vi "String Builder.vi"(9 "Omega":dbl, 10 "damping":dbl, 11 "A":dbl) -> (1 "a(t) string":string, 2 "v(t) string":string, 3 "x(t) string":string)   [LabVIEW 2019]
panel:
  out "Omega String":string
  out "damping string":string
  out "A string":string
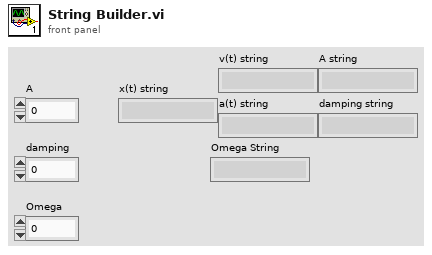
[diagram p1: front panel]
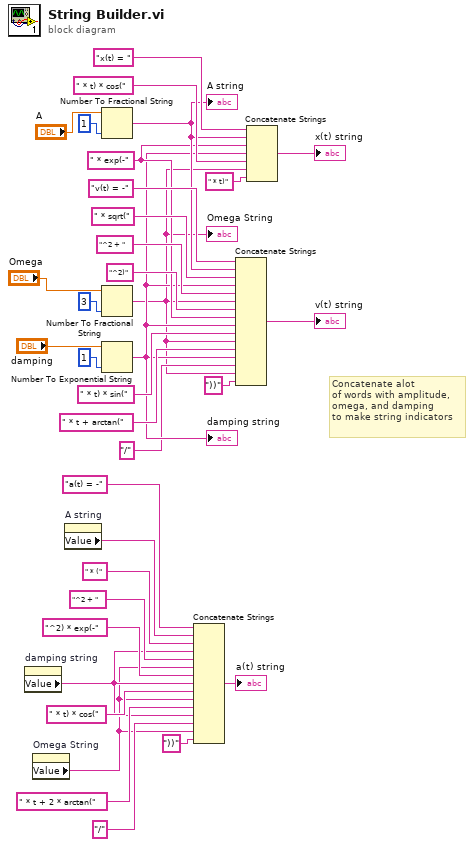
[diagram p0: block diagram]
diagram:
  w20 = " * exp(-"
  # "Concatenate alot\nof words with amplitude,\nomega, and damping\nto make string indicators"
  n1 = property on="damping string" class="Str"() -> ("Value"=w5:string)  [unwired: 2 in, 2 out]
  n2 = property on="Omega String" class="Str"() -> ("Value"=w3:string)  [unwired: 2 in, 2 out]
  n3 = property on="A string" class="Str"() -> ("Value"=w11:string)  [unwired: 2 in, 2 out]
  n4 = Number To Fractional String(number="A", precision (6)=i16 1) -> (F-format string=w24:string)  [unwired: 2 in]
  "A string" <- w24
  n5 = Number To Fractional String(number="Omega", precision (6)=i16 3) -> (F-format string=w15:string)  [unwired: 2 in]
  "Omega String" <- w15
  n6 = Number To Exponential String(number="damping", precision (6)=i16 1) -> (E-format string=w17:string)  [unwired: 2 in]
  "damping string" <- w17
  n7 = Concatenate Strings("a(t) = -" ("string"), w11, " * (" ("string"), w5, "^2 + " ("string"), w3, "^2) * exp(-" ("string"), w5, " * t) * cos(" ("string"), w3, " * t + 2 * arctan(" ("string"), w5, "/" ("string"), w3, "))" ("string")) -> (→"a(t) string":string)
  n8 = Concatenate Strings("v(t) = -" ("string"), w24, " * sqrt(" ("string"), w17, "^2 + " ("string"), w15, "^2)" ("string"), w20, w17, " * t) * sin(" ("string"), w15, " * t + arctan(" ("string"), w17, "/" ("string"), w15, "))" ("string")) -> (→"v(t) string":string)
  n9 = Concatenate Strings("x(t) = ", w24, w20, w17, " * t) * cos(", w15, " * t)") -> (→"x(t) string":string)
